vi "Charact One Point.vi"(0 "SG Path in":refnum<class "SG Abstract Path.lvclass">, 5 "Cal point in":T1, 11 "error in (no error)":errorcluster) -> (4 "SG Path out":refnum<class "SG Abstract Path.lvclass">, 15 "error out":errorcluster)   [LabVIEW 2023, in "RFFixtureCharact.Public.lvlib" / "SG Abstract Path.lvclass"]
uses:
  SG Abstract Path.lvclass
  C:/srd-semi-rfcal-software/AuxTools/STSRFFixtureCharactUtility/Source/Code Modules/Common/Base Classes/Path/Path.lvclass
  Scalar Path/Type Definitions/Cal Point.ctl
  Scalar Path/Type Definitions/Scalar Charact Result.ctl
  RFFixtureCharact.Public.lvlib
  Scalar Path/Scalar Path.lvclass
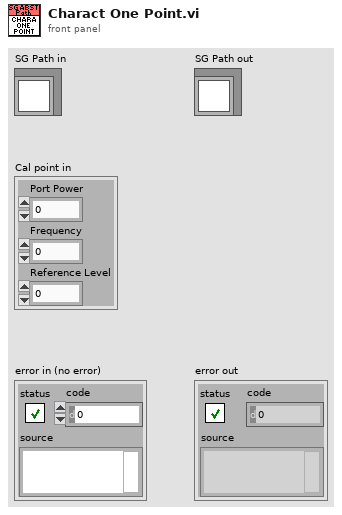
[diagram p1: front panel]
types:
  T1 = typedef "RFFixtureCharact.Public.lvlib/Scalar Path.lvclass/Cal Point.ctl" = cluster{"Port Power":dbl, "Frequency":dbl, "Reference Level":dbl}
  T2 = typedef "RFFixtureCharact.Public.lvlib/Scalar Path.lvclass/Scalar Charact Result.ctl" = cluster{"Port Power":dbl, "Reference Level":dbl, "Frequency":dbl, "Path Gain":dbl, "Out Of Limit":bool}
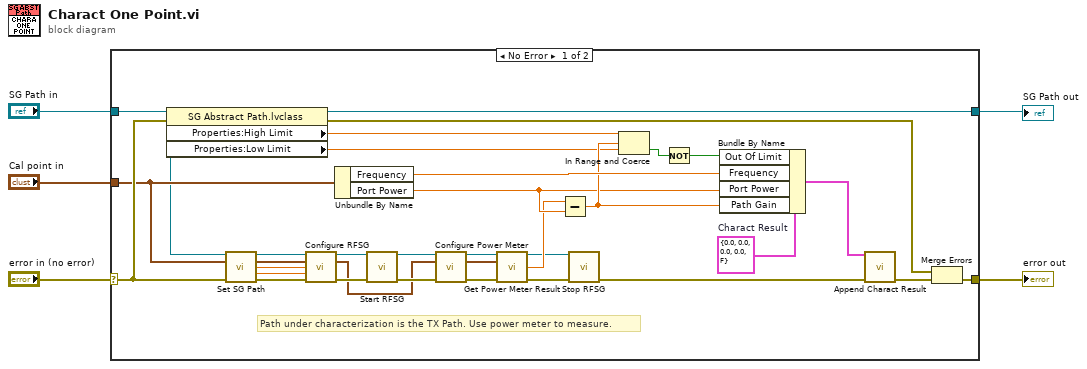
[diagram p0: block diagram]
diagram:
  n1 = case shown="No Error" "error in (no error)" {
    selector: "error in (no error)" -> [w26 w40]
    tunnel: "SG Path in" -> [w9 w39]
    tunnel: "Cal point in" -> [w16 _]
    tunnel: [w21 w40] -> w3
    tunnel: [w25 w39] -> w1
    frame No Error {
      w33 = T2 {"Port Power"=0.0, "Reference Level"=0.0, "Frequency"=0.0, "Path Gain"=0.0, "Out Of Limit"=FALSE}  # Charact Result
      # "Path under characterization is the TX Path. Use power meter to measure."
      n2 = property class="SG Abstract Path.lvclass"(reference=w9, error in=w26) -> (reference out=w25:refnum<class "SG Abstract Path.lvclass">, error out=w20:errorcluster, "Properties:High Limit"=w28:dbl, "Properties:Low Limit"=w27:dbl)
      n3 = call-dynamic "Set SG Path.vi"("Path in"=w9, "Cal point in"=w16, "error in (no error)"=w26) -> ("Path out"=w8:refnum<class "SG Abstract Path.lvclass">, "Cal point out"=w35:T1, "Source Gain"=w36:dbl, "Digital Gain"=w15:dbl, "error out"=w38:errorcluster)  [unwired: 8 in]
      n4 = call-dynamic "Configure RFSG.vi"("Path in"=w8, "Cal Point in"=w35, "External Gain"=w36, "Digital Gain"=w15, "error in (no error)"=w38) -> ("Path out"=w34:refnum<class "SG Abstract Path.lvclass">, "Cal Point out"=w12:T1, "error out"=w37:errorcluster)  [unwired: 8 in]
      n5 = Unbundle By Name(w16) -> ("Frequency"=w31:dbl, "Port Power"=w14:dbl)
      n6 = call-dynamic "Start RFSG.vi"("Path in"=w34, "error in (no error)"=w37) -> ("Path out"=w7:refnum<class "SG Abstract Path.lvclass">, "error out"=w13:errorcluster)  [unwired: 12 in]
      n7 = call-dynamic "Configure Power Meter.vi"("SG Path in"=w7, "Cal point in"=w12, "error in (no error)"=w13) -> ("SG Path out"=w17:refnum<class "SG Abstract Path.lvclass">, "Cal point out"=w11:T1, "error out"=w18:errorcluster)  [unwired: 10 in]
      n8 = call-dynamic "Get Power Meter Result.vi"("SG Path in"=w17, "Cal point in"=w11, "error in (no error)"=w18) -> ("SG Path out"=w6:refnum<class "SG Abstract Path.lvclass">, "Power (dBm)"=w10:dbl, "error out"=w19:errorcluster)  [unwired: 10 in]
      n9 = Subtract(x=w10, y=w14) -> (x-y=w29:dbl)
      n10 = call-dynamic "Stop RFSG.vi"("Path in"=w6, "error in (no error)"=w19) -> ("error out"=w24:errorcluster)  [unwired: 12 in, 1 out]
      n11 = In Range and Coerce(upper limit=w28, x=w29, lower limit=w27) -> (In Range?=w30:bool)  [unwired: 1 out]
      n12 = Not(x=w30) -> (.not. x?=w32:bool)
      n13 = Bundle By Name(cluster=w33, "Out Of Limit"=w32, "Frequency"=w31, "Port Power"=w14, "Path Gain"=w29) -> (w22:T2)
      n14 = call "Append Charact Result.vi"("Path cal resut in"=w22, "error in (no error)"=w24) -> ("error out"=w23:errorcluster)  [unwired: 13 in]
      n15 = Merge Errors(w20, w23) -> (w21:errorcluster)
    }
    frame Error {
    }
  }
  "error out" <- w3
  "SG Path out" <- w1
